vi "Main.vi"(7 "Event Sources":T1, 8 "error in":errorcluster, 9 "Folder names":string[](array[string])=["StaARx#[PLC]StaATesterRxSignals", "StaATx#[PLC]StaATesterTxSignals"], 10 "Sequence Context In":refnum<k7>, 11 "OPC UA In":refnum<class "OPC UA.lvclass">) -> (0 "error out":errorcluster, 3 "OPC UA Out":refnum<class "OPC UA.lvclass">, 5 "Station":string="asdfasdf")   [LabVIEW 2021, in "OPC UA.lvclass"]
uses:
  OPC UA.lvclass
  <vilib>/OPCUA/controls/OPC UA Client Refnum.ctl
  <vilib>/OPCUA/NI OPC UA Client.lvlib
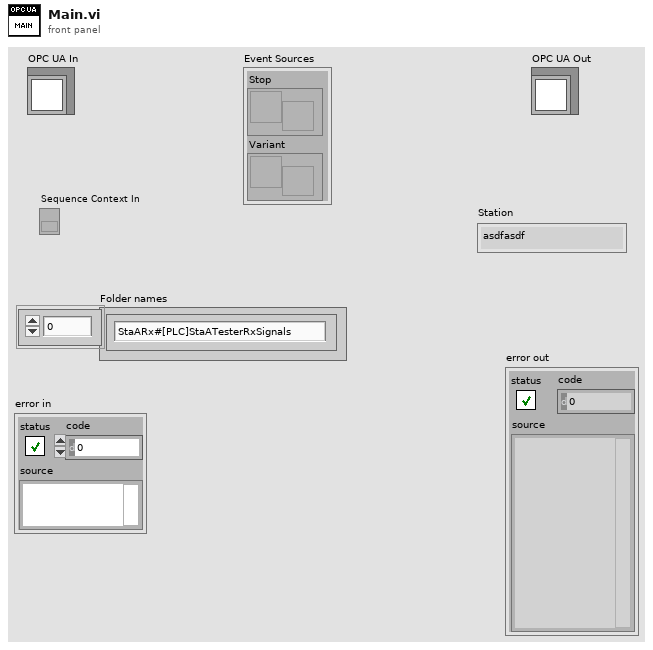
[diagram p1: front panel]
types:
  T1 = cluster{"Stop":refnum<user-event>, "Variant":refnum<user-event>}
  T2 = typedef "OPC UA Client Refnum.ctl" = refnum<k21>
  T3 = typedef "Subscription ID.ctl" = u32
  T4 = typedef "TestStand - Status Monitor.ctl" = cluster{"Sequence Context":refnum<k7>, "Execution":refnum<k7>, "Termination Monitor":refnum<k7>}
  T5 = cluster{"Event Registration Refnum":refnum<event-registration>, "Event Registration Refnum":refnum<event-registration>}
  T6 = typedef "Subscription Data Change.ctl" = cluster{"node ID":T7, " value":variant, "timestamp":timestamp, "data type":T8, "status code":T9}
  T7 = typedef "NodeId.ctl" = string
  T8 = typedef "Data Type.ctl" = u16
  T9 = typedef "OPC UA StatusCode.ctl" = u32
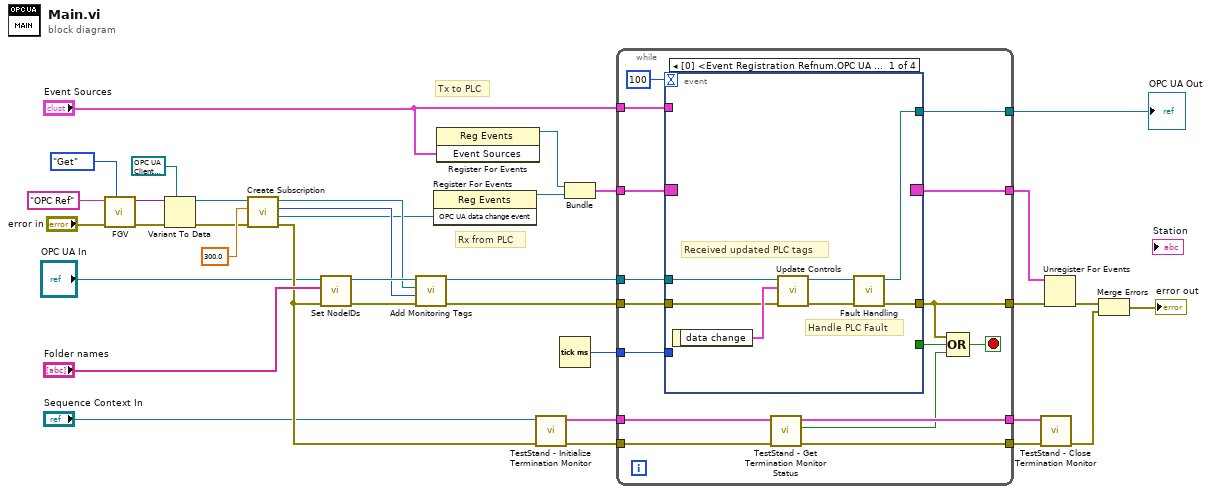
[diagram p0: block diagram]
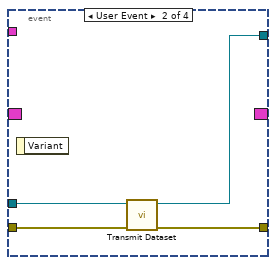
[diagram p2: hidden frame]
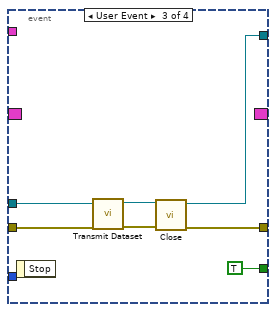
[diagram p3: hidden frame]
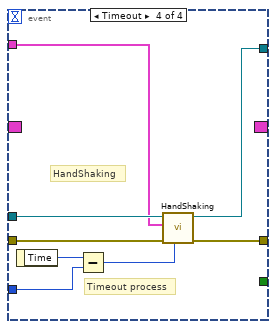
[diagram p4: hidden frame]
diagram:
  # "Tx to PLC"
  # "Rx from PLC"
  n1 = call "FGV.vi"("Method (Get)"=enum16{"Get", "Set"}."Get", "error in"="error in", "Name"="OPC Ref") -> ("error out"=w7:errorcluster, "Data out"=w6:variant)  [unwired: 7 in]
  n2 = Variant To Data(error in=w7, type=T2 refnum ("OPC UA client refnum out"), Variant=w6) -> (data=w33:T2, error out=w32:errorcluster)
  n3 = call <vilib>:"Create Subscription.vi"("error in (no error)"=w32, "publishing interval (1000 ms)"=300.0, "OPC UA client refnum in"=w33) -> ("error out"=w11:errorcluster, "OPC UA data change event"=w23:refnum<user-event>, "subscription ID out"=w27:T3, "OPC UA client refnum out"=w28:T2)  [unwired: 4 in, 1 out]
  n4 = call "Set NodeIDs.vi"("error in (no error)"=w11, "Folder names"="Folder names", "OPC UA in"="OPC UA In") -> ("error out"=w30:errorcluster, "OPC UA out"=w29:refnum<class "OPC UA.lvclass">)  [unwired: 7 in]
  n5 = call "Add Monitoring Tags.vi"("error in (no error)"=w30, "subscription ID"=w27, "OPC UA client refnum"=w28, "OPC UA in"=w29) -> ("error out"=w4:errorcluster, "OPC UAout"=w3:refnum<class "OPC UA.lvclass">)  [unwired: 6 in]
  n6 = register-events(w23) -> (reference out=w17:refnum<event-registration>)  [unwired: 2 in, 1 out]
  n7 = register-events("Event Sources") -> (reference out=w16:refnum<event-registration>)  [unwired: 2 in, 1 out]
  n8 = call <vilib>:"TestStand - Initialize Termination Monitor.vi"("error in (no error)"=w11, "Sequence Context In"="Sequence Context In") -> ("error out"=w25:errorcluster, "Status Monitor Out"=w24:T4)  [unwired: 8 in]
  n9 = Tick Count (ms)() -> (millisecond timer value=w15:u32)
  n10 = Bundle("Event Registration Refnum"=w16, "Event Registration Refnum"=w17) -> (w26:T5)  [unwired: 1 in]
  n11 = while {
    tunnel: w26 -> [w51]
    tunnel: w3 -> [w50]
    tunnel: w4 -> [w49]
    tunnel: [w37] -> w20
    tunnel: [w47] -> w19
    tunnel: w25 -> [w46]
    tunnel: w24 -> [w45]
    tunnel: [w43] -> w22
    tunnel: [w42] -> w21
    tunnel: "Event Sources" -> [w41]
    tunnel: [w40] -> w14
    tunnel: w15 -> [w39]
    stop <- w44 stop-if-true
    n12 = event shown="[0] <Event Registration Refnum.OPC UA data change event>: User Event" {
      selector: w51 -> [_ _ _ _]
      dyn-events: [_ _ _ _] -> w47
      timeout: 100 -> [_ _ _ _]
      tunnel: w50 -> [w58 w60 w67 w75]
      tunnel: w49 -> [w56 w61 w66 w74]
      tunnel: [w54 w62 w69 w77] -> w37
      tunnel: w41 -> [_ _ _ w70]
      tunnel: [w53 w59 w68 w76] -> w40
      tunnel: w39 -> [_ _ _ w72]
      tunnel: [_ _ TRUE ("Stop") _] -> w36
      event User Event {
        # "Handle PLC Fault"
        # "Received updated PLC tags"
        n13 = event-data() -> ("data change"=w57:T6[])  [unwired: 1 in]
        n14 = call "Update Controls.vi"("error in (no error)"=w56, "data change"=w57, "OPC UA in"=w58) -> ("error out"=w55:errorcluster, "OPC UA out"=w52:refnum<class "OPC UA.lvclass">)  [unwired: 7 in]
        n15 = call-dynamic "Fault Handling.vi"("error in (no error)"=w55, "OPC UA in"=w52) -> ("error out"=w54:errorcluster, "OPC UA out"=w53:refnum<class "OPC UA.lvclass">)  [unwired: 8 in]
      }
      event User Event {
        n16 = event-data() -> ()  [unwired: 1 in, 1 out]
        n17 = call "Transmit Dataset.vi"("error in (no error)"=w61, "OPC UA in"=w60) -> ("error out"=w62:errorcluster, "OPC UA out"=w59:refnum<class "OPC UA.lvclass">)  [unwired: 8 in]
      }
      event User Event {
        n18 = event-data() -> ()  [unwired: 1 in, 1 out]
        n19 = call "Transmit Dataset.vi"("error in (no error)"=w66, "OPC UA in"=w67) -> ("error out"=w64:errorcluster, "OPC UA out"=w65:refnum<class "OPC UA.lvclass">)  [unwired: 8 in]
        n20 = call-dynamic "Close.vi"("error in (no error)"=w64, "OPC UA in"=w65) -> ("error out"=w69:errorcluster, "OPC UA out"=w68:refnum<class "OPC UA.lvclass">)  [unwired: 8 in]
      }
      event Timeout {
        # "HandShaking"
        # "Timeout process"
        n21 = event-data() -> ("Time"=w73:u32)  [unwired: 1 in]
        n22 = Subtract(x=w73, y=w72) -> (x-y=w71:u32)
        n23 = call-dynamic "HandShaking.vi"("Elapsed Time"=w71, "error in (no error)"=w74, "Event Sources"=w70, "OPC UA in"=w75) -> ("error out"=w77:errorcluster, "OPC UA out"=w76:refnum<class "OPC UA.lvclass">)  [unwired: 6 in]
      }
    }
    n24 = call <vilib>:"TestStand - Get Termination Monitor Status.vi"("error in (no error)"=w46, "Status Monitor In"=w45) -> ("error out"=w43:errorcluster, "Terminating or Aborting"=w38:bool, "Status Monitor Out"=w42:T4)  [unwired: 7 in]
    n25 = Compound Arithmetic op=OR(w37, w36, w38) -> (w44:bool)
  }
  "OPC UA Out" <- w14
  n26 = call <vilib>:"TestStand - Close Termination Monitor.vi"("error in (no error)"=w22, "Status Monitor In"=w21) -> ("error out"=w12:errorcluster)  [unwired: 9 in]
  n27 = Unregister For Events(event registration refnum=w19, error in=w20) -> (error out=w13:errorcluster)
  n28 = Merge Errors(w13, w12) -> (→"error out":errorcluster)
